vi "GRPCClientExample.vi"() -> ()   [LabVIEW 2019, in "MicronGRPCClient.lvclass"]
uses:
  MicronGRPCClient.lvclass
  Base/Client/Typedefs/ServiceDetails.ctl
  Base/Client/MicronClient.lvclass
  <vilib>/SLL Toolkit/SLL File IO/SLL File IO.lvlib
panel:
  in  "Timeout (ms)":i32=-1
  in  "Connection Type":enum32{"Start New", "Connect Existing"}(tab)=enum."Connect Existing"
  in  "Path":path
  in  "Port":i32=50051
  in  "Fully Qualified Name (Optional)":string
  in  "UI":string(combo)="show"
  in  "Connection String":string="localhost:50051"
  in  "Fully Qualified Name (Optional)":string
  out "error out":errorcluster
  out "Response":string
  in  "Command":string="Hello World!"
  in  "Payload":string="Popping in to say hi!"
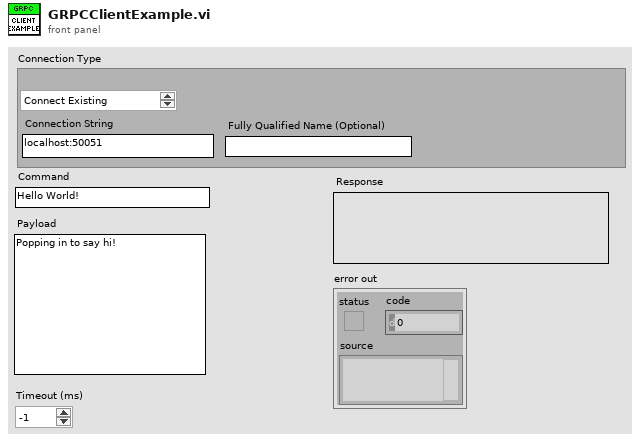
[diagram p1: front panel]
types:
  T1 = typedef "MicronClient.lvclass/ServiceDetails.ctl" = cluster{"Micron Path":path, "Network":string, "ServiceID":string, "Port":i32, "FullyQualifiedName":string, "UI":string, "Args":string, "Mode":string, "AutoRestartOnError?":bool}
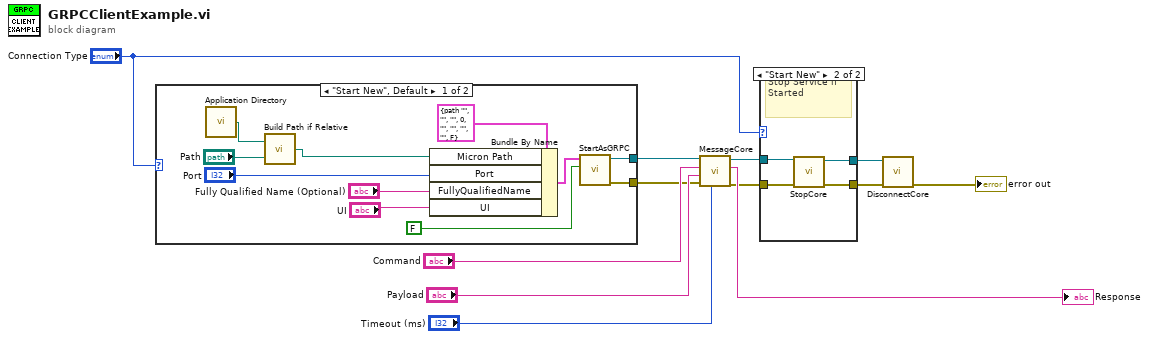
[diagram p0: block diagram]
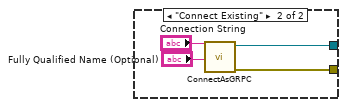
[diagram p3: hidden frame]
diagram:
  n1 = case shown="\"Start New\", Default" "Connection Type" {
    tunnel: [w23 w27] -> w8
    tunnel: [w22 w26] -> w7
    frame "Start New", Default {
      n2 = call <vilib>:"Application Directory.vi"() -> ("Application Directory"=w16:path)
      n3 = call <vilib>:"Build Path if Relative.vi"("Relative or Absolute Path"="Path", "Base Path"=w16) -> ("Path Out"=w17:path)
      n4 = Bundle By Name(cluster=T1 {"Micron Path"=path "", "Network"="", "ServiceID"="", "Port"=0, "FullyQualifiedName"="", "UI"="", "Args"="", "Mode"="", "AutoRestartOnError?"=FALSE} ("Service Details"), "Micron Path"=w17, "Port"="Port", "FullyQualifiedName"="Fully Qualified Name (Optional)", "UI"="UI") -> (w20:T1)
      n5 = call "StartAsGRPC.vi"("Simulate?"=FALSE, "Service Details"=w20) -> ("error out"=w23:errorcluster, "MicronClient out"=w22:refnum<class "MicronClient.lvclass">)  [unwired: 8 in]
    }
    frame "Connect Existing" {
      n6 = call "ConnectAsGRPC.vi"("Fully Qualified Name"="Fully Qualified Name (Optional)", "Connection String"="Connection String") -> ("error out"=w27:errorcluster, "MicronClient out"=w26:refnum<class "MicronClient.lvclass">)  [unwired: 8 in]
    }
  }
  n7 = call-dynamic "MessageCore.vi"("Timeout (ms)"="Timeout (ms)", "error in (no error)"=w8, "Payload"="Payload", "Command"="Command", "MicronClient in"=w7) -> ("error out"=w5:errorcluster, "Response"=→"Response":string, "MicronClient out"=w6:refnum<class "MicronClient.lvclass">)  [unwired: 4 in]
  n8 = case shown="\"Start New\"" "Connection Type" {
    tunnel: w6 -> [w29 w33]
    tunnel: w5 -> [w28 w32]
    tunnel: [w28 w31] -> w4
    tunnel: [w29 w30] -> w3
    frame Default {
    }
    frame "Start New" {
      # "Stop Service if Started"
      n9 = call-dynamic "StopCore.vi"("error in (no error)"=w32, "MicronClient in"=w33) -> ("error out"=w31:errorcluster, "MicronClient out"=w30:refnum<class "MicronClient.lvclass">)  [unwired: 7 in, 1 out]
    }
  }
  n10 = call-dynamic "DisconnectCore.vi"("error in (no error)"=w4, "MicronClient in"=w3) -> ("error out"=→"error out":errorcluster)  [unwired: 8 in, 1 out]
